vi "DataCNT-IsValid.vi"(8 "error in (no error)":errorcluster, 11 "DataCNT":T1) -> (0 "error out":errorcluster, 2 "Valid DataCNT?":bool, 3 "DataCNT(dup)":T1)   [LabVIEW 2017, in "Data Container.lvlib"]
uses:
  Data Container.lvlib
  TypeDef/Def-DataCNT.ctl
  TypeDef/Def-DataCNT Ico.ctl
panel:
  # "Connector Pane"
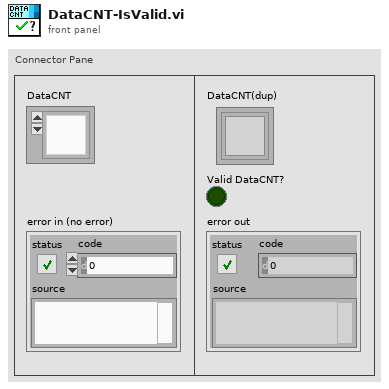
[diagram p1: front panel]
types:
  T1 = typedef "Data Container.lvlib/Def-DataCNT.ctl" = refnum<k1>
  T2 = typedef "Data Container.lvlib/Def-DataCNT DVR.ctl" = refnum<data-value>
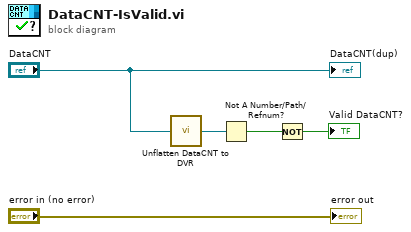
[diagram p0: block diagram]
diagram:
  n1 = call "Unflatten DataCNT to DVR.vi"("Data Contianer"="DataCNT") -> ("DataCNT DVR"=w1:T2)
  n2 = Not A Number/Path/Refnum?(number/path/refnum=w1) -> (NaN/Path/Refnum?=w4:bool)
  n3 = Not(x=w4) -> (.not. x?=→"Valid DataCNT?":bool)
  "error out" <- "error in (no error)"
  "DataCNT(dup)" <- "DataCNT"
